vi "Multiple UE9 Efunction Loop Example.vi"() -> (0 "error out A":errorcluster)   [LabVIEW 2021]
panel:
  in  "ConnectionType B":u16(ring) items=["LJ_ctUSB", "LJ_ctETHERNET"]
  in  "Address B":string="2"
  in  "ConnectionType A":u16(ring) items=["LJ_ctUSB", "LJ_ctETHERNET"]
  in  "Address A":string="1"
  out "FIO1 State In B":bool
  in  "DAC0 Voltage B":dbl format="%.3f"
  in  "FIO0 State Out B":bool
  out "Error Message B":string
  out "error out B":errorcluster
  out "AIN0 Voltage B":dbl format="%.6f"
  in  "stop":bool
  in  "Interval (ms)":u32=500
  out "FIO1 State In A":bool
  in  "DAC0 Voltage A":dbl format="%.3f"
  in  "FIO0 State Out A":bool
  out "Error Message A":string
  out "AIN0 Voltage A":dbl format="%.6f"
  # "Specify an IP address for Ethernet, or Local ID\nfor USB.  If FirstFound is selected, Local ID is\nignored for USB."
  # "UE9 with LocalID=1:  Sets DAC0, sets FIO0,\nreads AIN0, and reads FIO1."
  # "Specify an IP address for Ethernet, or Local ID\nfor USB.  If FirstFound is selected, Local ID is\nignored for USB."
  # "UE9 with LocalID=2:  Sets DAC0, sets FIO0,\nreads AIN0, and reads FIO1."
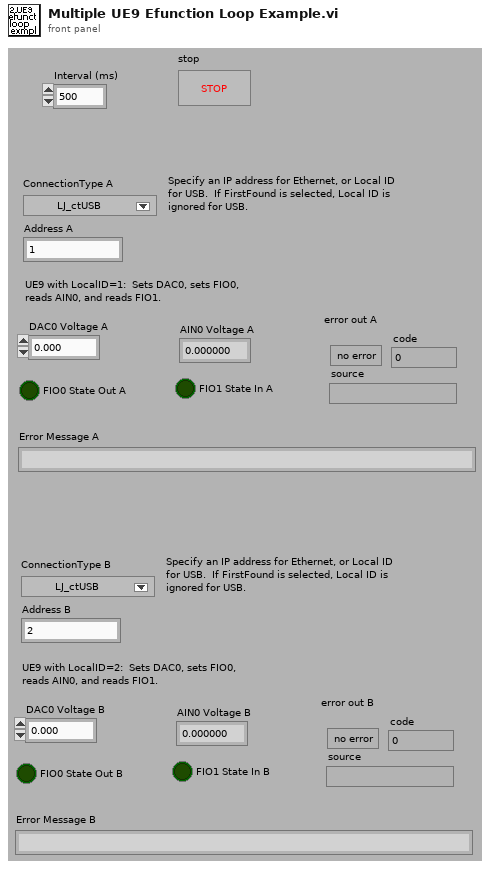
[diagram p1: front panel]
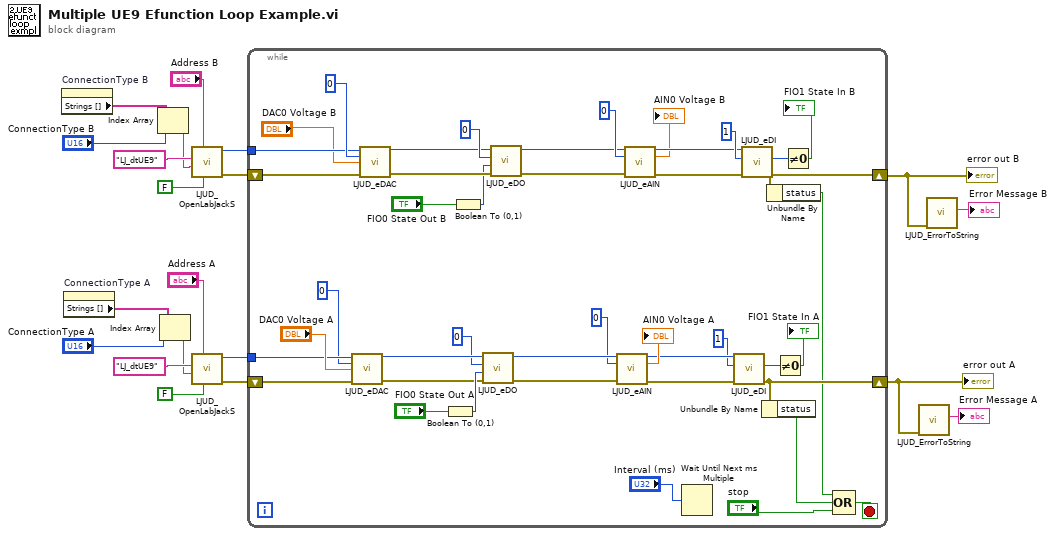
[diagram p0: block diagram]
diagram:
  n1 = property on="ConnectionType B" class="Ring (strict)"() -> ("Strings []"=w10:string[])  [unwired: 2 in, 2 out]
  n2 = property on="ConnectionType A" class="Ring (strict)"() -> ("Strings []"=w12:string[])  [unwired: 2 in, 2 out]
  n3 = Index Array(array=w10, index="ConnectionType B") -> (element=w8:string)
  n4 = Index Array(array=w12, index="ConnectionType A") -> (element=w7:string)
  n5 = call "LJUD_OpenLabJackS.vi"("FirstFound"=FALSE, "Address"="Address B", "ConnectionType"=w8, "DeviceType"="LJ_dtUE9") -> ("error out"=w3:errorcluster, "Handle"=w4:i32)  [unwired: 5 in, 1 out]
  n6 = call "LJUD_OpenLabJackS.vi"("FirstFound"=FALSE, "Address"="Address A", "ConnectionType"=w7, "DeviceType"="LJ_dtUE9") -> ("error out"=w1:errorcluster, "Handle"=w2:i32)  [unwired: 5 in, 1 out]
  n7 = while {
    shift-left: w3 -> [w43]
    shift-right: [w23] -> w13
    tunnel: w4 -> [w33]
    shift-left: w1 -> [w44]
    shift-right: [w45] -> w18
    tunnel: w2 -> [w57]
    stop <- w21 stop-if-true
    n8 = call "LJUD_eDAC.vi"("Handle In"=w57, "Channel"=0, "Voltage"="DAC0 Voltage A", "error in"=w44) -> ("Handle Out"=w55:i32, "error out"=w56:errorcluster)  [unwired: 10 in]
    n9 = call "LJUD_eDAC.vi"("Handle In"=w33, "Channel"=0, "Voltage"="DAC0 Voltage B", "error in"=w43) -> ("Handle Out"=w35:i32, "error out"=w34:errorcluster)  [unwired: 10 in]
    n10 = Boolean To (0,1)(Boolean="FIO0 State Out A") -> (0, 1=w61:i16)
    n11 = Boolean To (0,1)(Boolean="FIO0 State Out B") -> (0, 1=w31:i16)
    n12 = call "LJUD_eDO.vi"("error in"=w56, "State"=w61, "Channel"=0, "Handle In"=w55) -> ("error out"=w54:errorcluster, "Handle Out"=w53:i32)  [unwired: 6 in]
    n13 = call "LJUD_eDO.vi"("error in"=w34, "State"=w31, "Channel"=0, "Handle In"=w35) -> ("error out"=w36:errorcluster, "Handle Out"=w37:i32)  [unwired: 6 in]
    n14 = call "LJUD_eAIN.vi"("Handle In"=w53, "ChannelP"=0, "error in"=w54) -> ("Handle Out"=w49:i32, "Voltage"=→"AIN0 Voltage A":dbl, "error out"=w58:errorcluster)  [unwired: 10 in]
    n15 = call "LJUD_eAIN.vi"("Handle In"=w37, "ChannelP"=0, "error in"=w36) -> ("Handle Out"=w41:i32, "Voltage"=→"AIN0 Voltage B":dbl, "error out"=w32:errorcluster)  [unwired: 10 in]
    n16 = Wait Until Next ms Multiple(millisecond multiple="Interval (ms)") -> ()  [unwired: 1 out]
    n17 = call "LJUD_eDI.vi"("error in"=w58, "Channel"=1, "Handle In"=w49) -> ("error out"=w45:errorcluster, "State"=w62:i32)  [unwired: 6 in, 1 out]
    n18 = call "LJUD_eDI.vi"("error in"=w32, "Channel"=1, "Handle In"=w41) -> ("error out"=w23:errorcluster, "State"=w30:i32)  [unwired: 6 in, 1 out]
    n19 = Unbundle By Name(w45) -> ("status"=w25:bool)
    n20 = Unbundle By Name(w23) -> ("status"=w22:bool)
    n21 = Not Equal To 0?(x=w62) -> (x != 0?=→"FIO1 State In A":bool)
    n22 = Not Equal To 0?(x=w30) -> (x != 0?=→"FIO1 State In B":bool)
    n23 = Compound Arithmetic op=OR(w22, w25, "stop") -> (w21:bool)
  }
  "error out A" <- w18
  "error out B" <- w13
  n24 = call "LJUD_ErrorToString.vi"("error in"=w18) -> ("String"=→"Error Message A":string)  [unwired: 10 in]
  n25 = call "LJUD_ErrorToString.vi"("error in"=w13) -> ("String"=→"Error Message B":string)  [unwired: 10 in]
